vi "Exit mode.vi"(8 "error in (no error)":errorcluster, 11 "VISA resource name":refnum<visa-resource-name>) -> (0 "error out":errorcluster, 3 "VISA resource name out":refnum<visa-resource-name>)   [LabVIEW 2017, in "ScientiFic DC Power Supply.lvlib"]
doc: "Queries the current instrument firmware revision and instrument driver revision.\n\nRefer to the Readme file for detailed driver information including modification history."
uses:
  ScientiFic DC Power Supply.lvlib
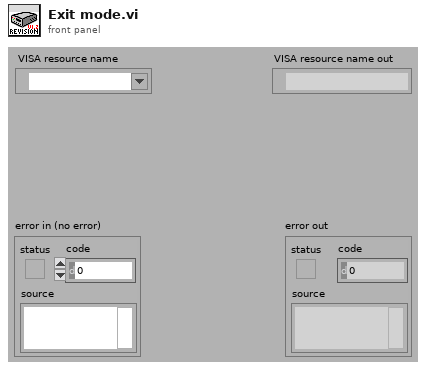
[diagram p1: front panel]
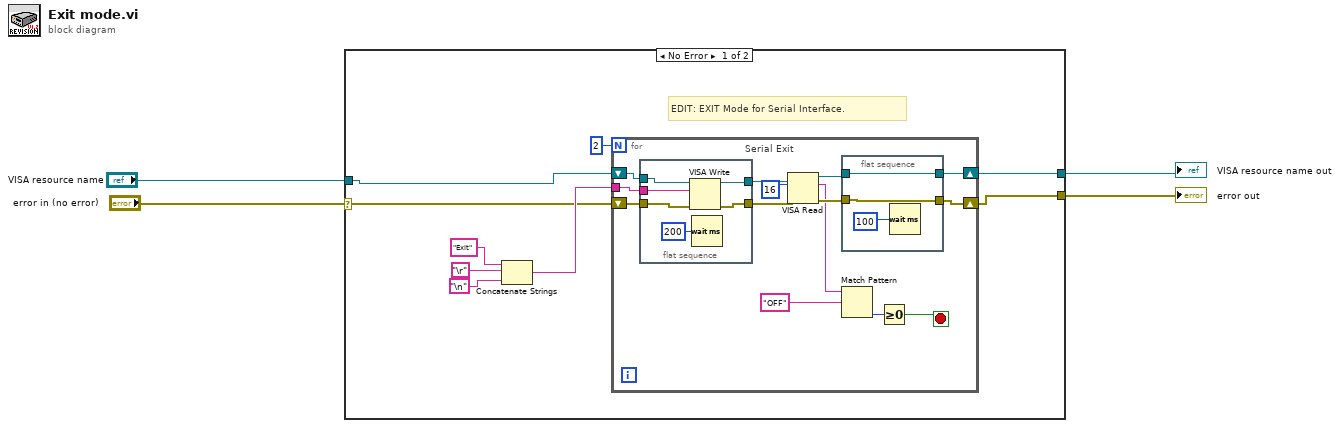
[diagram p0: block diagram]
diagram:
  n1 = case shown="No Error" "error in (no error)" {
    selector: "error in (no error)" -> [w5 w37]
    tunnel: "VISA resource name" -> [w13 w38]
    tunnel: [w7 w38] -> w3
    tunnel: [w6 w37] -> w2
    frame No Error {
      # "EDIT: EXIT Mode for Serial Interface."
      n2 = Concatenate Strings("Exit" ("string"), "\r", "\n") -> (w8:string)
      n3 = for {
        N: 2 -> [_]
        tunnel: w8 -> [w18]
        shift-right: [w19] -> w6
        shift-left: w5 -> [w27]
        shift-right: [w20] -> w7
        shift-left: w13 -> [w26]
        stop <- w15 stop-if-true
        # "Serial Exit"
        n4 = flat-sequence {
          tunnel: w27 -> [w33]
          tunnel: w26 -> [w32]
          tunnel: [w31] -> w25
          tunnel: [w30] -> w24
          tunnel: w18 -> [w29]
          frame #0 {
            n5 = VISA Write(VISA resource name=w32, write buffer=w29, error in (no error)=w33) -> (VISA resource name out=w30:refnum<visa-resource-name>, error out=w31:errorcluster)  [unwired: 1 out]
            n6 = Wait (ms)(milliseconds to wait=u32 200) -> ()  [unwired: 1 out]
          }
        }
        n7 = VISA Read(VISA resource name=w24, byte count=u32 16, error in (no error)=w25) -> (VISA resource name out=w22:refnum<visa-resource-name>, read buffer=w17:string, error out=w21:errorcluster)  [unwired: 1 out]
        n8 = flat-sequence {
          tunnel: w22 -> [w35]
          tunnel: w21 -> [w34]
          tunnel: [w35] -> w20
          tunnel: [w34] -> w19
          frame #0 {
            n9 = Wait (ms)(milliseconds to wait=u32 100) -> ()  [unwired: 1 out]
          }
        }
        n10 = Match Pattern(string=w17, regular expression="OFF") -> (offset past match=w16:i32)  [unwired: 1 in, 3 out]
        n11 = Greater Or Equal To 0?(x=w16) -> (x >= 0?=w15:bool)
      }
    }
    frame Error {
    }
  }
  "VISA resource name out" <- w3
  "error out" <- w2
